vi "sedSpectrometer_getEvent_LargeFileObjectAvailable.vi"(8 "error in (no error)":errorcluster, 11 "logevent_LargeFileObjectAvailable_Ctl":T1) -> (0 "error out":errorcluster, 2 "function return":i32, 3 "logevent_LargeFileObjectAvailable_Ctl out":T1)   [LabVIEW 2016, in "SALLV_sedSpectrometer.lvlib"]
doc: "int sedSpectrometer_shm_getEvent_LargeFileObjectAvailableLV(sedSpectrometer_logevent_LargeFileObjectAvailableLV *logevent_LargeFileObjectAvailable_Ctl );"
uses:
  SALLV_sedSpectrometer.lvlib
  DataTypes/logevent_LargeFileObjectAvailable.ctl
  SALLV_sedSpectrometer.so
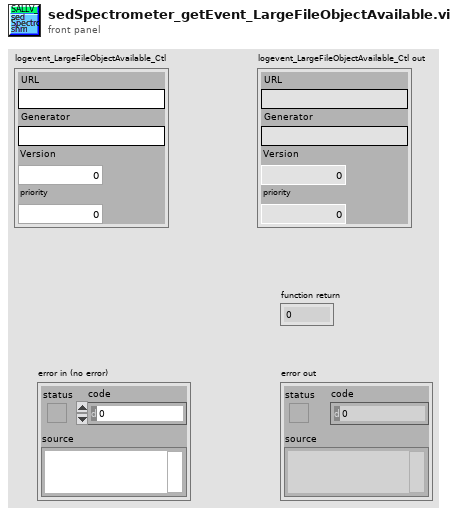
[diagram p1: front panel]
types:
  T1 = typedef "SALLV_sedSpectrometer.lvlib/logevent_LargeFileObjectAvailable.ctl" = cluster{"URL":string, "Generator":string, "Version":sgl, "priority":i32}
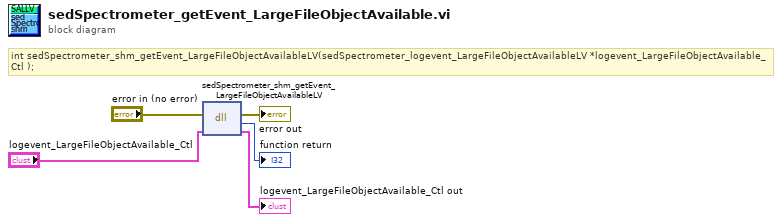
[diagram p0: block diagram]
diagram:
  # "int sedSpectrometer_shm_getEvent_LargeFileObjectAvailableLV(sedSpectrometer_logevent_LargeFileObjectAvailableLV *logevent_LargeFileObjectAvailable_Ctl );"
  n1 = dll-call lib="home/harini/TCS/SALLV_sedSpectrometer/SALLV_sedSpectrometer.*" fn="sedSpectrometer_shm_getEvent_LargeFileObjectAvailableLV"(error in="error in (no error)", "logevent_LargeFileObjectAvailable_Ctl"="logevent_LargeFileObjectAvailable_Ctl") -> (error out=→"error out":errorcluster, →"function return":i32, "logevent_LargeFileObjectAvailable_Ctl"=→"logevent_LargeFileObjectAvailable_Ctl out":T1)  [unwired: 2 in, 1 out]
